vi "Remove Language.vi"(8 "error in (no error)":errorcluster, 11 "Controller in":refnum<class "Controller.lvclass">) -> (0 "error out":errorcluster, 3 "Controller out":refnum<class "Controller.lvclass">)   [LabVIEW 2013, in "SET Project Editor.lvlib" / "Controller.lvclass"]
uses:
  Controller.lvclass
  Controller.lvclass/Controller.ctl
  SET Project Data/Project Data Class/Project Data.lvclass
  SET Project Data/Resource Data Class/Resource Data.lvclass/Resource Data.ctl
  <vilib>/ActorFramework/Message Enqueuer/Message Enqueuer.lvclass/Message Enqueuer.ctl
  SET Project Data/Resource Data Class/Read Languages.vi
  <vilib>/ActorFramework/Message Enqueuer/Enqueue.vi
  <vilib>/ActorFramework/Message Priority Queue/Priority Enqueue.vi
  SET Project Data/Resource Data Class/Resource Data.lvclass
  UI View Messages/UI Refresh Data Msg/UI Refresh Data Msg.lvclass
  SET Project Editor.lvlib
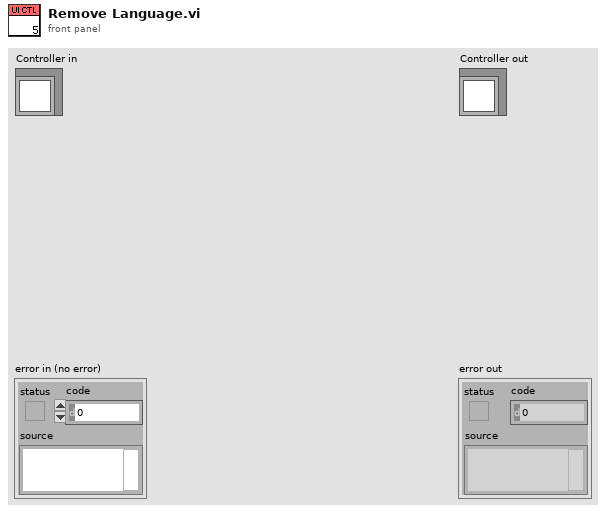
[diagram p1: front panel]
types:
  T1 = typedef "SET Project Data.lvlib/ProjFile_Language Data.ctl" = cluster{"Tag":string, "Name":string, "Code Page":u16}
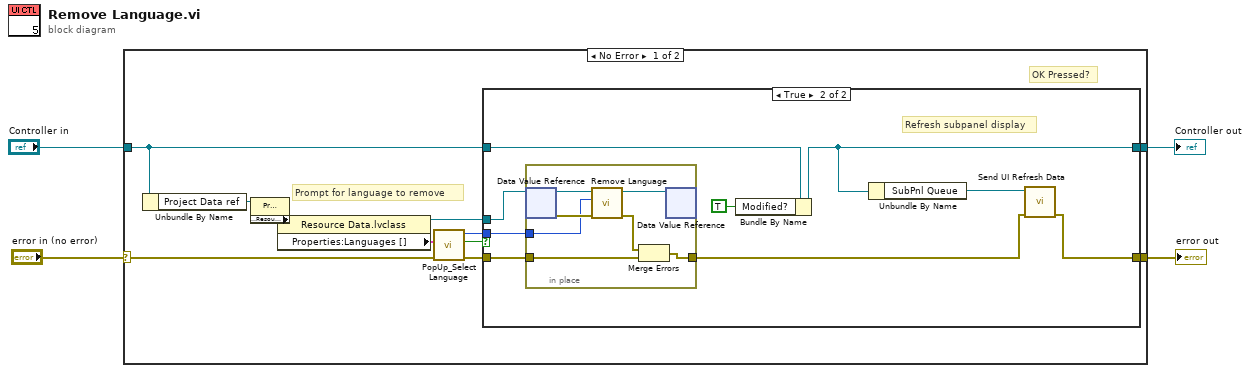
[diagram p0: block diagram]
diagram:
  n1 = case shown="No Error" "error in (no error)" {
    selector: "error in (no error)" -> [w6 w35]
    tunnel: [w14 w35] -> w1
    tunnel: [w15 w34] -> w2
    tunnel: "Controller in" -> [w12 w34]
    frame No Error {
      # "Prompt for language to remove"
      # "OK Pressed?"
      n2 = Unbundle By Name(w12) -> ("Project Data ref"=w9:refnum<data-value>)
      n3 = property class="Project Data.lvclass"(reference=w9) -> ("Properties:Resource Data ref"=w8:refnum<data-value>)  [unwired: 1 in, 2 out]
      n4 = property class="Resource Data.lvclass"(reference=w8) -> (reference out=w5:refnum<data-value>, "Properties:Languages []"=w7:T1[])  [unwired: 1 in, 1 out]
      n5 = call "PopUp_Select Language.vi"("error in (no error)"=w6, "Languages"=w7) -> ("error out"=w13:errorcluster, "OK Pressed?"=w11:bool, "LangIndex"=w10:i32)  [unwired: 7 in]
      n6 = case shown="True" w11 {
        tunnel: [w17 w21] -> w15
        tunnel: [w16 w19] -> w14
        tunnel: w13 -> [w16 w26]
        tunnel: w12 -> [w17 w23]
        tunnel: w10 -> [_ w25]
        tunnel: w5 -> [_ w24]
        frame False {
        }
        frame True {
          # "Refresh subpanel display"
          n7 = in-place {
            in-place-border: w26 -> [w31]
            in-place-border: [w30] -> w18
            in-place-border: w25 -> [w27]
            n8 = in-place-dvr #1(w24) -> (w33:refnum<class "Resource Data.lvclass">, w32:errorcluster)
            n9 = call "Remove Language.vi"("error in (no error)"=w32, "index"=w27, "LangFile in"=w33) -> ("error out"=w29:errorcluster, "LangFile out"=w28:refnum<class "Resource Data.lvclass">)  [unwired: 7 in]
            n10 = Merge Errors(w29, w31) -> (w30:errorcluster)
            n11 = in-place-dvr #1(w28) -> ()  [unwired: 2 out]
          }
          n12 = Bundle By Name(cluster=w23, "Modified?"=TRUE) -> (w21:refnum<class "Controller.lvclass">)
          n13 = Unbundle By Name(w21) -> ("SubPnl Queue"=w20:refnum<class "Message Enqueuer.lvclass">)
          n14 = call "Send UI Refresh Data.vi"("error in (no error)"=w18, "Message Enqueuer"=w20) -> ("error out"=w19:errorcluster)  [unwired: 8 in, 1 out]
        }
      }
    }
    frame Error {
    }
  }
  "error out" <- w1
  "Controller out" <- w2
